vi "MischerMonitor_Merge_Cluster.vi"(1 "Mischer  Control":T3, 2 "Mischer  Status":T2) -> (0 "Mischer Monitor":T1)   [LabVIEW 2019]
uses:
  Mischer/Mischer-Control.ctl
  Mischer/Mischer-Status.ctl
  Mischer/Mischer-Cluster.ctl
panel:
  # "2"
  # "to Condenser"
  # "1"
  # "7"
  # "From Still"
  # "5"
  # "Mischer\nEinheit"
  # "12"
  # "Cold\nTrap"
  # "Dump"
  # "9"
  # "8"
  # "2"
  # "to Condenser"
  # "1"
  # "7"
  # "From Still"
  # "5"
  # "Mischer\nEinheit"
  # "12"
  # "Cold\nTrap"
  # "Dump"
  # "9"
  # "8"
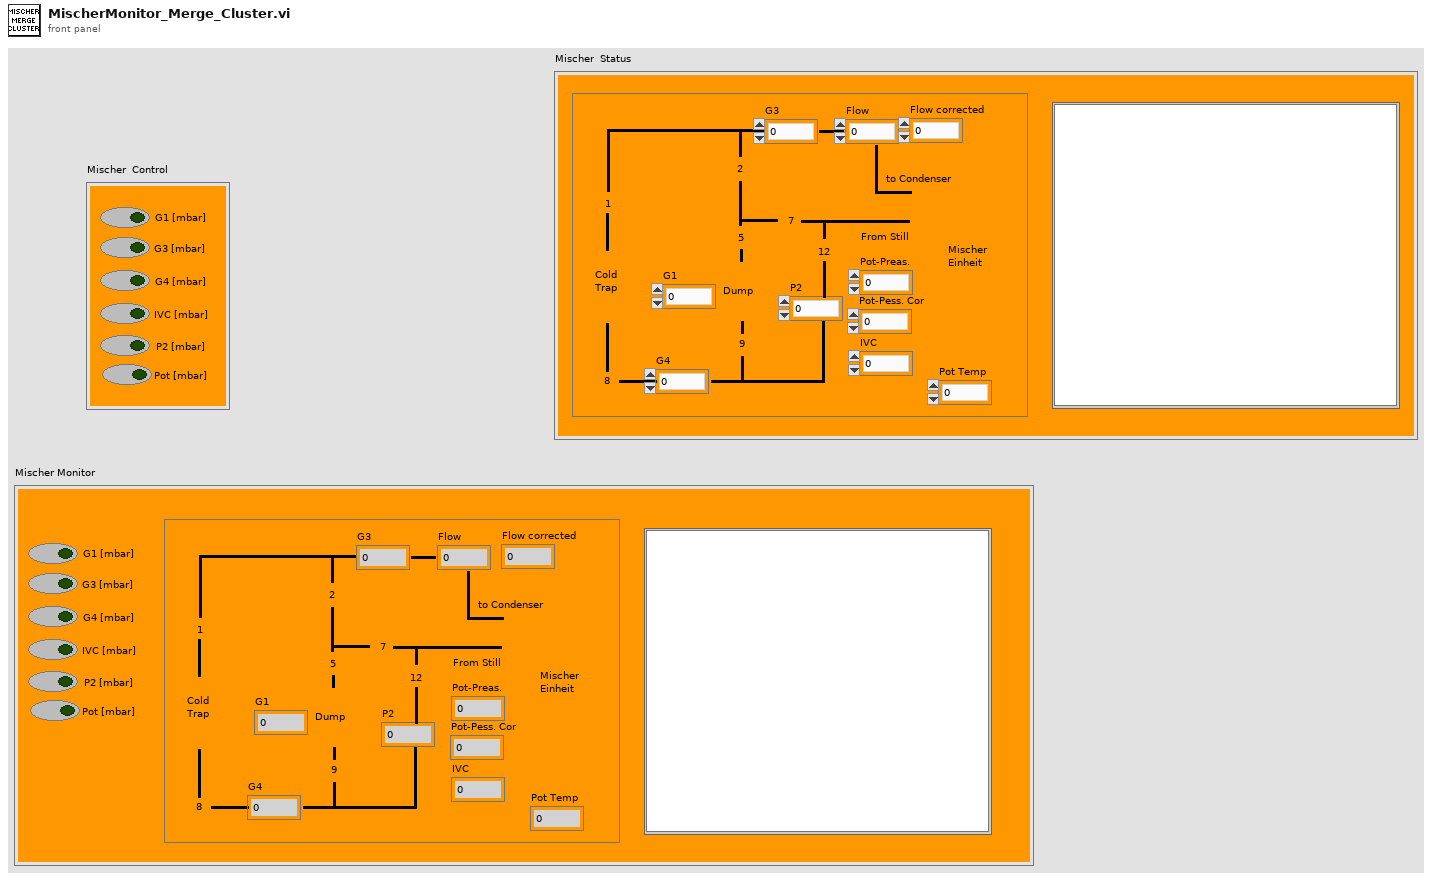
[diagram p1: front panel]
types:
  T1 = typedef "Mischer-Cluster.ctl" = cluster{"G4":dbl, "G1":dbl, "P2":dbl, "G3":dbl, "Flow":dbl, "Pot-Preas.":dbl, "IVC":dbl, "G1 [mbar]":bool, "G3 [mbar]":bool, "G4 [mbar]":bool, "IVC [mbar]":bool, "P2 [mbar] ":bool, "Flow corrected":dbl, "Pot-Pess. Cor":dbl, "Pot Temp":dbl, "Pot [mbar]":bool, "Plot":dbl[][]}
  T2 = typedef "Mischer-Status.ctl" = cluster{"G4":dbl, "G1":dbl, "P2":dbl, "G3":dbl, "Flow":dbl, "Pot-Preas.":dbl, "IVC":dbl, "Flow corrected":dbl, "Pot-Pess. Cor":dbl, "Pot Temp":dbl, "Plot":dbl[][]}
  T3 = typedef "Mischer-Control.ctl" = cluster{"G1 [mbar]":bool, "G3 [mbar]":bool, "G4 [mbar]":bool, "IVC [mbar]":bool, "P2 [mbar] ":bool, "Pot [mbar]":bool}
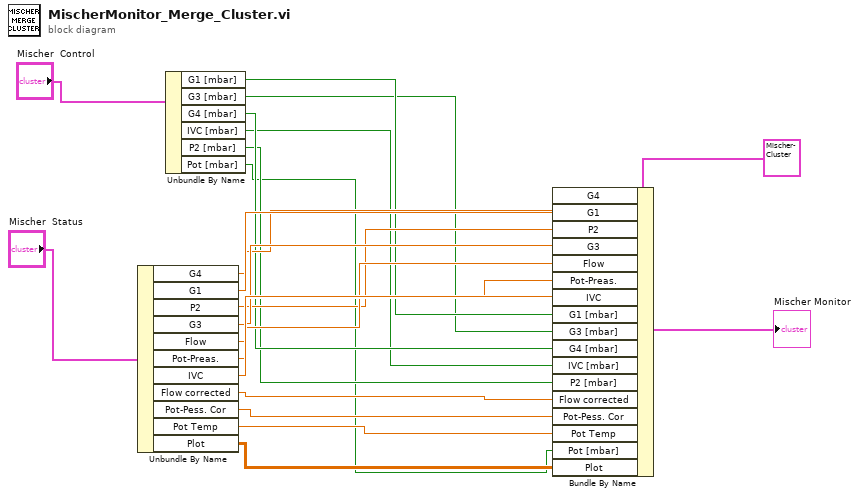
[diagram p0: block diagram]
diagram:
  n1 = Unbundle By Name("Mischer  Status") -> ("G4"=w7:dbl, "G1"=w8:dbl, "P2"=w9:dbl, "G3"=w10:dbl, "Flow"=w11:dbl, "Pot-Preas."=w12:dbl, "IVC"=w13:dbl, "Flow corrected"=w14:dbl, "Pot-Pess. Cor"=w15:dbl, "Pot Temp"=w16:dbl, "Plot"=w17:dbl[][])
  n2 = Unbundle By Name("Mischer  Control") -> ("G1 [mbar]"=w6:bool, "G3 [mbar]"=w5:bool, "G4 [mbar]"=w4:bool, "IVC [mbar]"=w3:bool, "P2 [mbar]"=w2:bool, "Pot [mbar]"=w1:bool)
  n3 = Bundle By Name(cluster=T1 {"G4"=0.0, "G1"=0.0, "P2"=0.0, "G3"=0.0, "Flow"=0.0, "Pot-Preas."=0.0, "IVC"=0.0, "G1 [mbar]"=FALSE, "G3 [mbar]"=FALSE, "G4 [mbar]"=FALSE, "IVC [mbar]"=FALSE, "P2 [mbar] "=FALSE, "Flow corrected"=0.0, "Pot-Pess. Cor"=0.0, "Pot Temp"=0.0, "Pot [mbar]"=FALSE, "Plot"=[]} ("Mischer Monitor"), "G4"=w7, "G1"=w8, "P2"=w9, "G3"=w10, "Flow"=w11, "Pot-Preas."=w12, "IVC"=w13, "G1 [mbar]"=w6, "G3 [mbar]"=w5, "G4 [mbar]"=w4, "IVC [mbar]"=w3, "P2 [mbar]"=w2, "Flow corrected"=w14, "Pot-Pess. Cor"=w15, "Pot Temp"=w16, "Pot [mbar]"=w1, "Plot"=w17) -> (→"Mischer Monitor":T1)
